vi "H5Pget_gc_references.vi"(6 "error in (no error)":errorcluster, 9 "HDF5 Property List Ref":T1) -> (0 "error out":errorcluster, 2 "Collect Reference Garbage":bool, 3 "HDF5 Property List Ref out":T1)   [LabVIEW 2017]
doc: "Returns garbage collecting references setting."
uses:
  <vilib>/UPVI/lvhdf5/library.llb/HDF5 Ref.ctl
  <vilib>/UPVI/lvhdf5/hdf5.dll
panel:
  # "LVHDF5 Toolkit\nCopyright (c) 2005-2013 by Jason D. Sommerville\nCopyright (c) 2014 by UPVI, LLC.\n\nThis use and distribution of this file is governed by the terms found in \nLICENSE.txt distributed with this toolkit and installed at\n <user.lib>\\_lvhdf5\\LICENSE.txt"
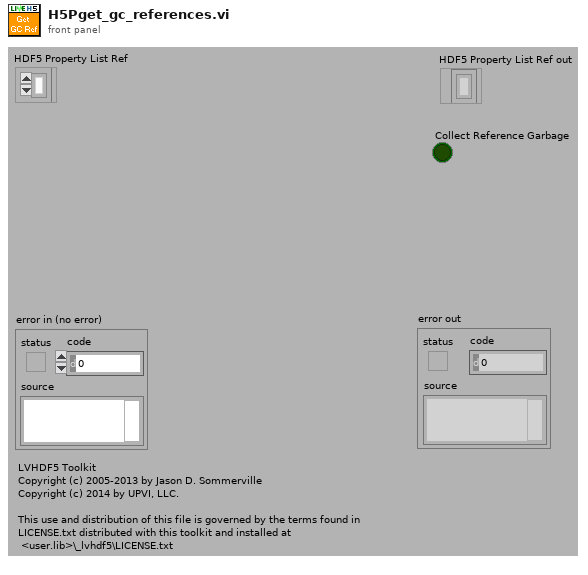
[diagram p1: front panel]
types:
  T1 = typedef "HDF5 Ref.ctl" = refnum<k1>
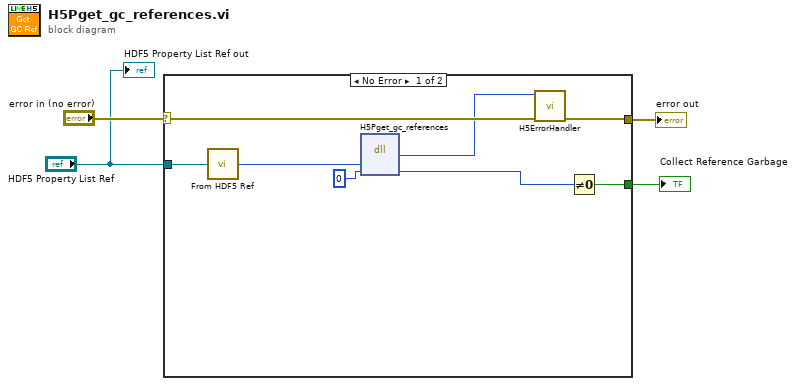
[diagram p0: block diagram]
diagram:
  n1 = case shown="No Error" "error in (no error)" {
    selector: "error in (no error)" -> [w12 w13]
    tunnel: [w11 w13] -> w3
    tunnel: "HDF5 Property List Ref" -> [w10 _]
    tunnel: [w5 _] -> w1
    frame No Error {
      n2 = call <vilib>:"From HDF5 Ref.vi"("HDF5 Ref"=w10) -> ("I32"=w9:i32)
      n3 = dll-call lib="C:/Program Files/National Instruments/LabVIEW 2017/vi.lib/UPVI/lvhdf5/hdf5.dll" fn="H5Pget_gc_references"("plist_id"=w9, "gc_ref"=u32 0) -> (w8:i32, "gc_ref"=w6:u32)  [unwired: 4 in, 2 out]
      n4 = call <vilib>:"H5ErrorHandler.vi"("error in (no error)"=w12, "herr_t"=w8) -> ("error out"=w11:errorcluster)  [unwired: 3 in, 4 out]
      n5 = Not Equal To 0?(x=w6) -> (x != 0?=w5:bool)
    }
    frame Error {
    }
  }
  "error out" <- w3
  "Collect Reference Garbage" <- w1
  "HDF5 Property List Ref out" <- "HDF5 Property List Ref"
